vi "generate graph.vi"(8 "error in (no error)":errorcluster, 11 "Waveform in":refnum<class "Waveform.lvclass">) -> (0 "error out":errorcluster, 2 "Mixed Signal Graph":T1(graph), 3 "Waveform out":refnum<class "Waveform.lvclass">)   [LabVIEW 2012, in "Waveform.lvclass"]
uses:
  Waveform.lvclass
  Waveform.lvclass/Waveform.ctl
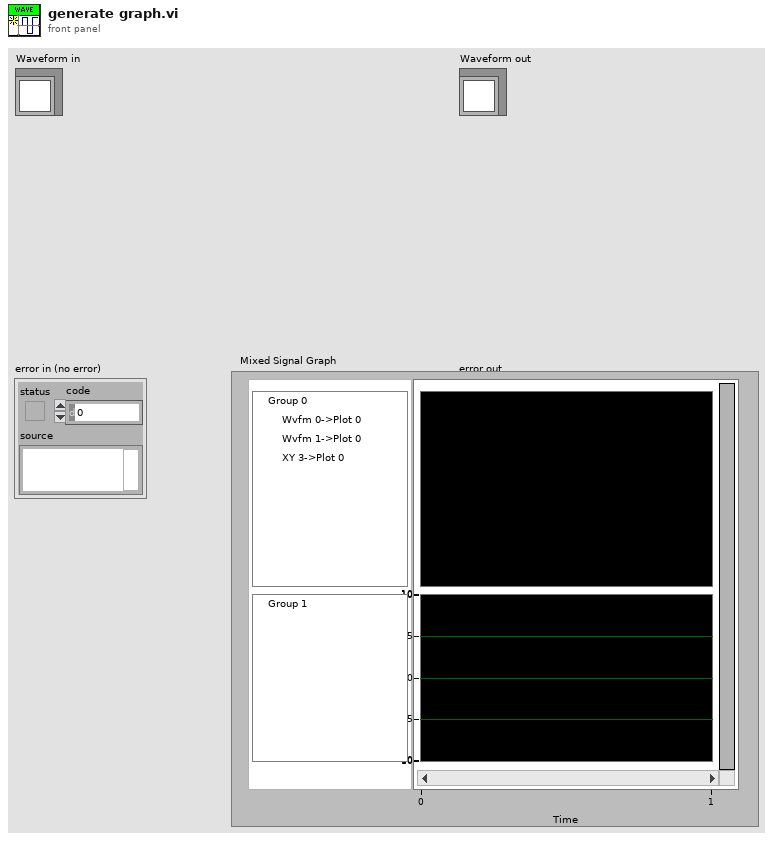
[diagram p1: front panel]
types:
  T1 = cluster{"galvo1 waveform":waveform(dbl), "galvo2 waveform":waveform(dbl), dbl[]}
  T2 = typedef "PC_wavelength.ctl" = dbl
  T3 = cluster{"galvo1 waveform":waveform(dbl), "galvo2 waveform":waveform(dbl), T2[]}
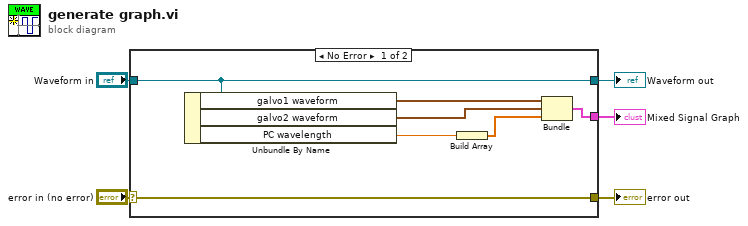
[diagram p0: block diagram]
diagram:
  n1 = case shown="No Error" "error in (no error)" {
    selector: "error in (no error)" -> [w8 w14]
    tunnel: [w8 w14] -> w4
    tunnel: [w12 w13] -> w2
    tunnel: "Waveform in" -> [w12 w13]
    tunnel: [w10 _] -> w1
    frame No Error {
      n2 = Unbundle By Name(w12) -> ("galvo1 waveform"=w11:waveform(dbl), "galvo2 waveform"=w9:waveform(dbl), "PC wavelength"=w7:T2)
      n3 = Build Array(w7) -> (w6:T2[])
      n4 = Bundle("galvo1 waveform"=w11, "galvo2 waveform"=w9, w6) -> (w10:T3)  [unwired: 1 in]
    }
    frame Error {
    }
  }
  "error out" <- w4
  "Waveform out" <- w2
  "Mixed Signal Graph" <- w1
